vi "StopSignal-StopAllInDefaultOrder.vi"(8 "error in (no error)":errorcluster, 9 "interval time(ms)":u32, 10 "reason(\"\")":string, 11 "Reverse？":bool) -> (0 "error out":errorcluster)   [LabVIEW 2017, in "StopSignal.lvlib"]
uses:
  StopSignal.lvlib
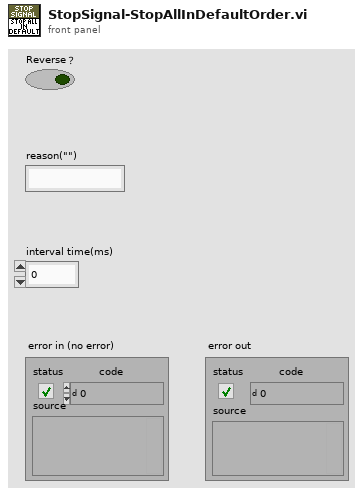
[diagram p1: front panel]
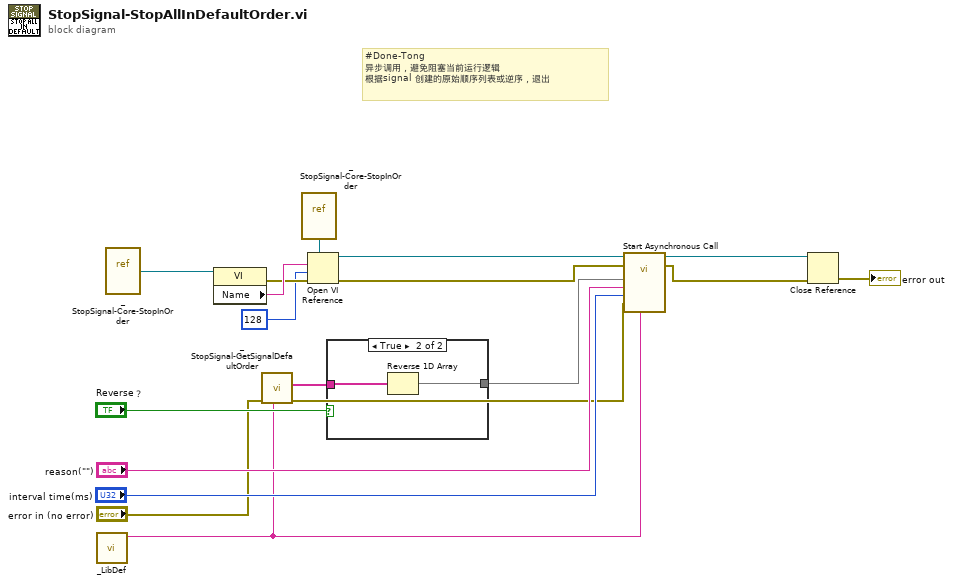
[diagram p0: block diagram]
diagram:
  # "#Done-Tong\n异步调用，避免阻塞当前运行逻辑\n根据signal 创建的原始顺序列表或逆序，退出"
  n1 = call "_LibDef.vi"() -> ("LIBNAME"=w1:string)  [unwired: 11 in]
  n2 = vi-ref "_StopSignal-Core-StopInOrder.vi"() -> (w16:refnum<vi>)
  n3 = property class="VI"(reference=w16) -> (error out=w17:errorcluster, "Name"=w18:string)  [unwired: 1 in, 1 out]
  n4 = call "_StopSignal-GetSignalDefaultOrder.vi"("LIBNAME"=w1, "error in (no error)"="error in (no error)") -> ("error out"=w4:errorcluster, "SignalInArray"=w3:string[])  [unwired: 8 in]
  n5 = vi-ref "_StopSignal-Core-StopInOrder.vi"() -> (w15:refnum<vi>)
  n6 = Open VI Reference(type specifier VI Refnum (for type only)=w15, vi path=w18, options=128, error in (no error)=w17) -> (vi reference=w14:refnum<vi>, error out=w13:errorcluster)  [unwired: 2 in]
  n7 = case shown="True" "Reverse？" {
    tunnel: w3 -> [w19 w21]
    tunnel: [w19 w20] -> w2
    frame False {
    }
    frame True {
      n8 = Reverse 1D Array(array=w21) -> (reversed array=w20:string[])
    }
  }
  n9 = call-by-ref "Start Asynchronous Call"(reference=w14, error in=w13, "LIBNAME"=w1, 8:"error in (no error)"=w4, "interval time(ms)"="interval time(ms)", "reason(\"\")"="reason(\"\")", "name(\"\")"=w2) -> (reference out=w11:refnum<vi>, error out=w12:errorcluster)  [unwired: 5 in, 2 out]
  n10 = Close Reference(reference=w11, error in (no error)=w12) -> (error out=→"error out":errorcluster)
